vi "test_Create Value Change & Trigger Message.vi"(8 "error in (no error)":errorcluster, 11 "TestCase in":refnum<class "Instrument Addon Scripting API Messages Unit Tests.lvclass">) -> (0 "error out":errorcluster, 3 "TestCase out":refnum<class "Instrument Addon Scripting API Messages Unit Tests.lvclass">)   [LabVIEW 2019, in "Instrument Addon Scripting API Messages Unit Tests.lvclass"]
uses:
  Instrument Addon Scripting API Messages Unit Tests.lvclass
  <vilib>/addons/_JKI Toolkits/VI Tester/TestCase.llb/TestCase.lvclass
  Instrument Addon Scripting API Test Assets/Instrument Addon Scripting API Test Assets.lvclass
  APIs/Scripting API/Instrument Addon Scripting API.lvlib
  NationalInstruments.VeriStand.SystemDefinitionAPI
  <vilib>/NI VeriStand/Custom Device Tools/Custom Device Utility Library/Custom Device Utility Library.lvlib
  Addon/Addon Shared/SubVIs/Constants.vi
  Addon/Addon Shared/Instrument Addon Shared.lvlib
  <vilib>/NI VeriStand/Custom Device Tools/Custom Device Utility Library/NI VeriStand - Search for Item by GUID.vi
  APIs/Scripting API/TypeDefs/Protection Types.ctl
  APIs/Scripting API/TypeDefs/Message Settings.ctl
  Addon/Addon Shared/Types/FG Control.ctl
  Addon/Addon Shared/Types/Message Generation Type.ctl
  APIs/Scripting API/Messages/Create Message - Value Change & Trigger.vi
  C:/Program Files (x86)/National Instruments/LabVIEW 2018/vi.lib/addons/_JKI Toolkits/VI Tester/TestCase.llb/TestCase.lvclass
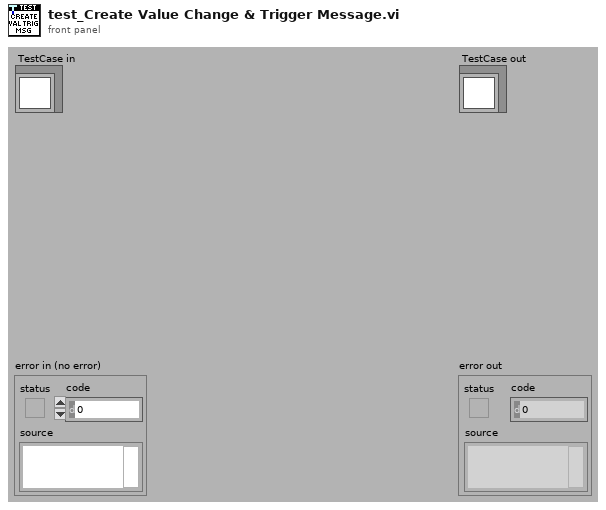
[diagram p1: front panel]
types:
  T1 = typedef "Instrument Addon Shared.lvlib/Message Generation Type.ctl" = enum16{"Trigger Only", "Periodic & Trigger", "Value Change & Trigger"}
  T2 = typedef "Instrument Addon Shared.lvlib/FG Control.ctl" = enum16{"Get", "Set"}
  T3 = typedef "Instrument Addon Scripting API.lvlib/Message Settings.ctl" = cluster{"Protection":T4, "Enable Periodic Default":bool, "Trigger Channel refnum":u64}
  T4 = typedef "Instrument Addon Scripting API.lvlib/Protection Types.ctl" = enum16{"None", "CRC-32", "Checksum U16", "Checksum U32", "Checksum U8"}
  T5 = typedef "Custom Device API.lvlib/Custom Device Item Ref.ctl" = u64
  T6 = typedef "Instrument Addon Shared.lvlib/Trigger Parameters.ctl" = cluster{"Use Channel":bool, "Channel Path":string}
  T7 = typedef "Instrument Addon Shared.lvlib/Message Parameters.ctl" = cluster{"Generation Type":T1, "Period":dbl, "Include Protection":bool, "Type":string}
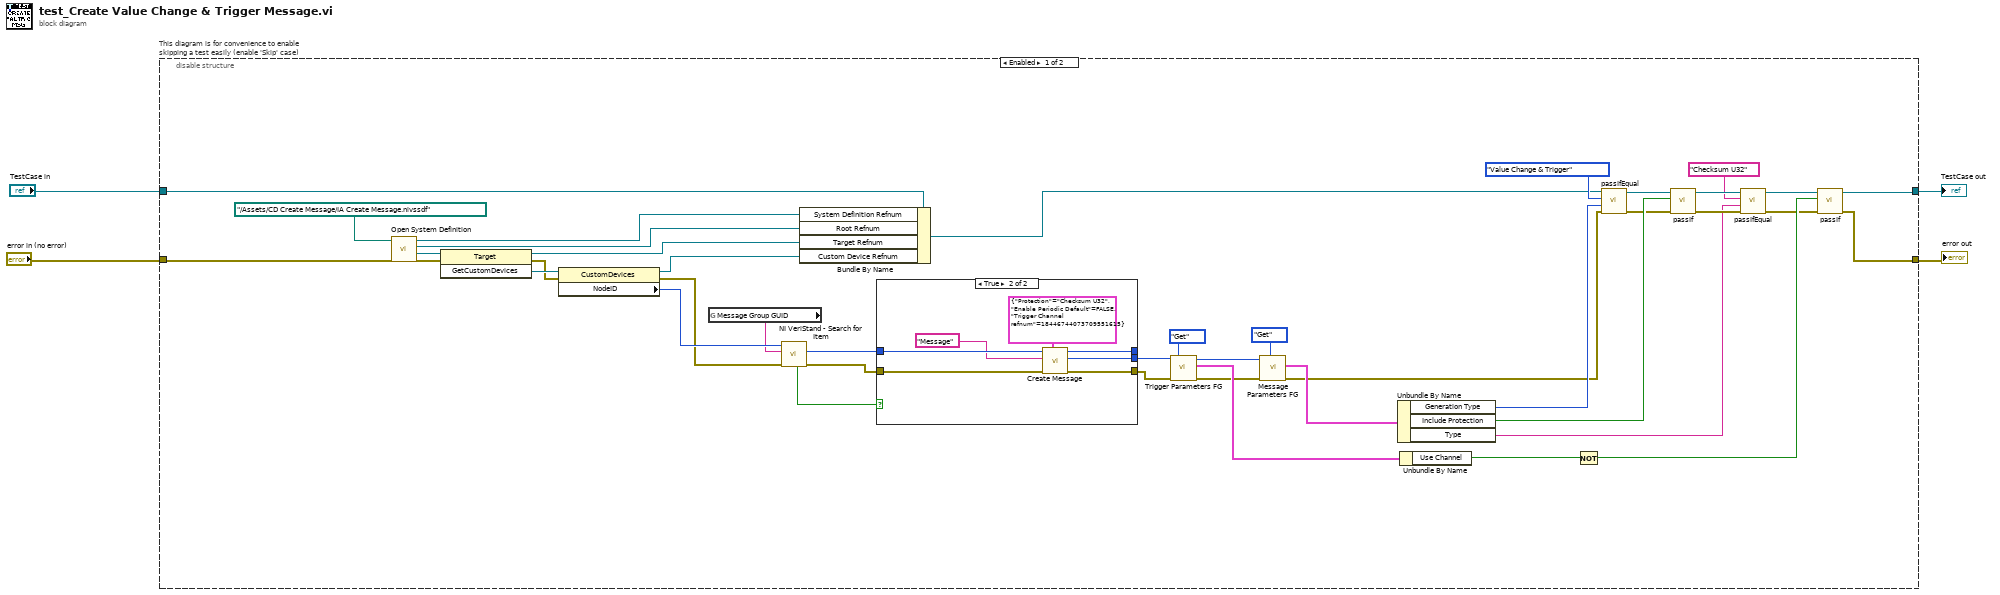
[diagram p0: block diagram]
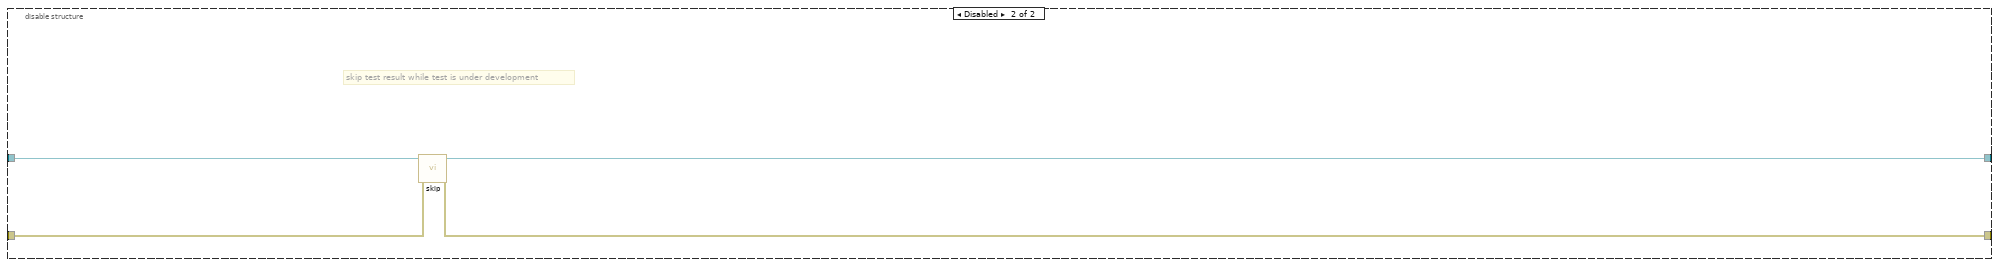
[diagram p3: hidden frame]
diagram:
  n1 = disable-structure "This diagram is for convenience to enable skipping a test easily (enable 'Skip' case)" shown="Enabled" {
    disable-tunnel: "TestCase in" -> [w10 w58]
    disable-tunnel: [w14 w56] -> w1
    disable-tunnel: [w13 w57] -> w3
    disable-tunnel: "error in (no error)" -> [w45 w55]
    frame Enabled {
      n2 = call "Open System Definition.vi"("error in (no error)"=w45, "System Definition File"=path "../Assets/CD Create Message/IA Create Message.nivssdf" ("SDF file")) -> ("error out"=w38:errorcluster, "Target Refnum"=w44:refnum<k24>, "Root Refnum"=w7:refnum<k24>, "System Definition Refnum"=w8:refnum<k24>)  [unwired: 6 in]
      n3 = invoke class="Target" method="GetCustomDevices"(reference=w44, error in=w38) -> (reference out=w6:refnum<k24>, error out=w37:errorcluster, "GetCustomDevices"=w43:refnum<k24>)  [unwired: 1 in]
      n4 = property class="CustomDevices"(reference=w43, error in=w37) -> (reference out=w5:refnum<k24>, error out=w36:errorcluster, "NodeID"=w42:u64)
      n5 = global read "Constants.vi" "Message Group GUID"() -> (w41:string)
      n6 = call-poly <vilib>:"NI VeriStand - Search for Item.vi"("error in"=w36, "Item GUID"=w41, "Section Ref in"=w42) -> ("error out"=w35:errorcluster, "Item Ref"=w40:T5, "Found"=w39:bool)  [unwired: 5 in, 1 out]
      n7 = Bundle By Name(cluster=w10, "System Definition Refnum"=w8, "Root Refnum"=w7, "Target Refnum"=w6, "Custom Device Refnum"=w5) -> (w9:refnum<class "Instrument Addon Scripting API Messages Unit Tests.lvclass">)
      n8 = case shown="True" w39 {
        tunnel: w40 -> [_ w54]
        tunnel: [w47 w53] -> w15
        tunnel: w35 -> [w47 w52]
        tunnel: [_ w51] -> w12
        tunnel: [_ w50] -> _
        frame False {
        }
        frame True {
          n9 = call-poly "Create Message.vi"("optional settings"=T3 {"Protection"=enum."Checksum U32", "Enable Periodic Default"=FALSE, "Trigger Channel refnum"=18446744073709551615} ("Message Settings"), "error in (no error)"=w52, "message name"="Message", "message group refnum in"=w54) -> ("error out"=w53:errorcluster, "message refnum out"=w51:T5, "message group refnum out"=w50:T5)  [unwired: 5 in]
        }
      }
      n10 = call "Trigger Parameters FG.vi"("Action"=FG_Control."Get", "error in (no error)"=w15, "Item Ref in"=w12) -> ("error out"=w20:errorcluster, "Trigger Parameters"=w22:T6, "Item Ref out"=w19:T5)  [unwired: 6 in]
      n11 = call "Message Parameters FG.vi"("Action"=FG_Control."Get", "error in (no error)"=w20, "Item Ref in"=w19) -> ("error out"=w21:errorcluster, "Message Settings out"=w23:T7)  [unwired: 6 in, 1 out]
      n12 = Unbundle By Name(w23) -> ("Generation Type"=w26:T1, "Include Protection"=w29:bool, "Type"=w30:string)
      n13 = Unbundle By Name(w22) -> ("Use Channel"=w33:bool)
      n14 = Not(x=w33) -> (.not. x?=w34:bool)
      n15 = call-dynamic "passIfEqual.vi"("error in (no error)"=w21, "y"=w26, "x"=Message_Generation_Type."Value Change & Trigger" ("Generation Type"), "TestCase in"=w9) -> ("error out"=w27:errorcluster, "TestCase out"=w28:refnum<class "Instrument Addon Scripting API Messages Unit Tests.lvclass">)  [unwired: 6 in]
      n16 = call-dynamic "passIf.vi"("error in (no error)"=w27, "pass"=w29, "TestCase in"=w28) -> ("error out"=w31:errorcluster, "TestCase out"=w32:refnum<class "Instrument Addon Scripting API Messages Unit Tests.lvclass">)  [unwired: 7 in]
      n17 = call-dynamic "passIfEqual.vi"("error in (no error)"=w31, "y"=w30, "x"="Checksum U32" ("Type"), "TestCase in"=w32) -> ("error out"=w25:errorcluster, "TestCase out"=w24:refnum<class "Instrument Addon Scripting API Messages Unit Tests.lvclass">)  [unwired: 6 in]
      n18 = call-dynamic "passIf.vi"("error in (no error)"=w25, "pass"=w34, "TestCase in"=w24) -> ("error out"=w13:errorcluster, "TestCase out"=w14:refnum<class "Instrument Addon Scripting API Messages Unit Tests.lvclass">)  [unwired: 7 in]
    }
    frame Disabled {
      # "skip test result while test is under development"
      n19 = call <vilib>:"skip.vi"("error in (no error)"=w55, "TestCase in"=w58) -> ("error out"=w57:errorcluster, "TestCase out"=w56:refnum<class "Instrument Addon Scripting API Messages Unit Tests.lvclass">)  [unwired: 8 in]
    }
  }
  "error out" <- w3
  "TestCase out" <- w1
